vi "countrate.vi"() -> ()   [LabVIEW 2015]
uses:
  <vilib>/platform/TimedLoop/XDataNode/XDataNode.xnode
  <vilib>/Platform/TimedLoop/XDataNode/nitl_modes.ctl
  <vilib>/Platform/TimedLoop/XDataNode/XDNodeRunTimeDep.lvlib
  <vilib>/Platform/TimedLoop/XDataNode/wakeup.ctl
  <vilib>/Platform/TimedLoop/XDataNode/timing_clust.ctl
panel:
  out "counts per second":dbl(knob) scale=0.0..100.0
  in  "stop":bool
  # "Demo count rate VI for Physics 434"
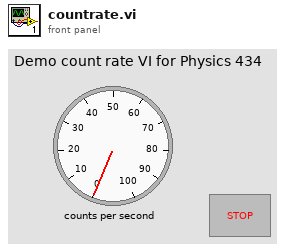
[diagram p1: front panel]
types:
  T1 = typedef "XDNodeRunTimeDep.lvlib/timing_clust.ctl" = cluster{"Expected End [f-1]":u64, "Actual End [f-1]":u64, "Finished Late? [f-1]":bool, "Expected End [i-1]":u64, "Actual End [i-1]":u64, "Finished Late? [i-1]":bool, "Expected Start [i]":u64, "Actual Start [i]":u64, "Expected Start [f]":u64, "Actual Start [f]":u64, "Source Name":string, "Structure Name":string, "Period":i64, "Deadline":i64, "Offset":i64, "Start":i64, "Priority":i32, "Timeout":i32, "Mode":T2, "Wakeup Reason":T3, "Error":errorcluster, "Source Type":string, "Secondary Source Type":string, "Global End Time":u64, "Global Start Time":u64, "Frame Duration":u64, "Iteration Duration":u64, "Assigned CPU":i32, "I/O Scan Engine Mode":u32}
  T2 = typedef "XDNodeRunTimeDep.lvlib/nitl_modes.ctl" = enum32{"No Change", "Process missed periods, maintain original phase", "Discard missed periods, maintain original phase", "Process missed periods, ignore original phase", "Discard missed periods, ignore original phase"}
  T3 = typedef "XDNodeRunTimeDep.lvlib/wakeup.ctl" = enum32{"Normal", "Aborted", "Asynchronous wakeup", "Timing source error", "Timed loop error", "Timeout"}
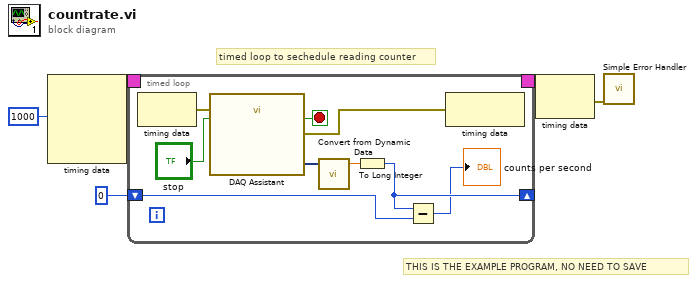
[diagram p0: block diagram]
diagram:
  # "THIS IS THE EXAMPLE PROGRAM, NO NEED TO SAVE"
  # "timed loop to sechedule reading counter"
  n1 = node-c288(i64 1000 ("Period")) -> (w5:T1)  [unwired: 3 in]
  n2 = timed-loop {
    timing: w5 -> [_]
    timing-out: [_] -> w4
    shift-right: [w10] -> _
    shift-left: 0 -> [w13]
    stop <- w12 stop-if-true
    n3 = node-c288() -> (w6:errorcluster)  [unwired: 1 in]
    n4 = call "DAQ Assistant"("error in"=w6, "stop (F)"="stop") -> ("data"=w14:dynamicdata, "stopped"=w12:bool, "error out"=w7:errorcluster)  [unwired: 14 in, 1 out]
    n5 = call "Convert from Dynamic Data"("Dynamic Data Type"=w14) -> ("Scalar"=w8:dbl)  [unwired: 3 in]
    n6 = To Long Integer(number=w8) -> (32bit integer=w10:i32)
    n7 = Subtract(x=w10, y=w13) -> (x-y=→"counts per second":i32)
    n8 = node-c288(w7) -> ()  [unwired: 1 out]
  }
  n9 = node-c288(w4) -> (w1:errorcluster)
  n10 = call <vilib>:"Simple Error Handler.vi"("error in (no error)"=w1) -> ()  [unwired: 4 in, 5 out]
